vi "testOpenCloseVeriStandConnection.vi"(8 "error in (no error)":errorcluster, 11 "TestCase in":refnum<class "VeriStandTestCaseSystemTests.lvclass">) -> (0 "error out":errorcluster, 3 "TestCase out":refnum<class "VeriStandTestCaseSystemTests.lvclass">)   [LabVIEW 2016, in "VeriStandTestCaseSystemTests.lvclass"]
uses:
  VeriStandTestCaseSystemTests.lvclass
  VeriStandTestUtilities/SystemDefinitionInformation.ctl
  VeriStandTestUtilities/TargetInformation.ctl
  VeriStandTestUtilities/ChassisInformation.ctl
  <vilib>/NI Veristand/Execution/Workspace/WorkspaceAPI.ctl
  NationalInstruments.VeriStand.ClientAPI
  VeriStandTestCase.lvclass
  <vilib>/addons/_JKI Toolkits/VI Tester/TestCase.llb/TestCase.lvclass
  C:/Program Files (x86)/National Instruments/LabVIEW 2016/vi.lib/addons/_JKI Toolkits/VI Tester/TestCase.llb/TestCase.lvclass
  VeriStandTestUtilities/VeriStandTestUtilities.lvlib
  <vilib>/NI VeriStand/Execution/Workspace/NI_VS Workspace ExecutionAPI.lvlib
panel:
  out "WorkspaceManager":T1
  out "System Definition Information":T2
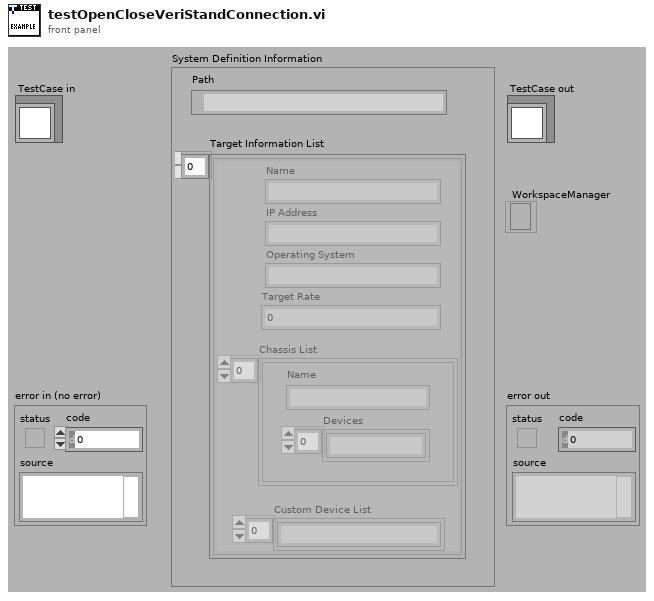
[diagram p1: front panel]
types:
  T1 = typedef "NI_VS Workspace ExecutionAPI.lvlib/WorkspaceAPI.ctl" = refnum<k24>
  T2 = typedef "VeriStandTestUtilities.lvlib/SystemDefinitionInformation.ctl" = cluster{"Path":path, "Target Information List":T3[]}
  T3 = typedef "VeriStandTestUtilities.lvlib/TargetInformation.ctl" = cluster{"Name":string, "IP Address":string, "Operating System":string, "Target Rate":dbl, "Chassis List":T4[], "Custom Device List":string[]}
  T4 = typedef "VeriStandTestUtilities.lvlib/ChassisInformation.ctl" = cluster{"Name":string, "Devices":string[]}
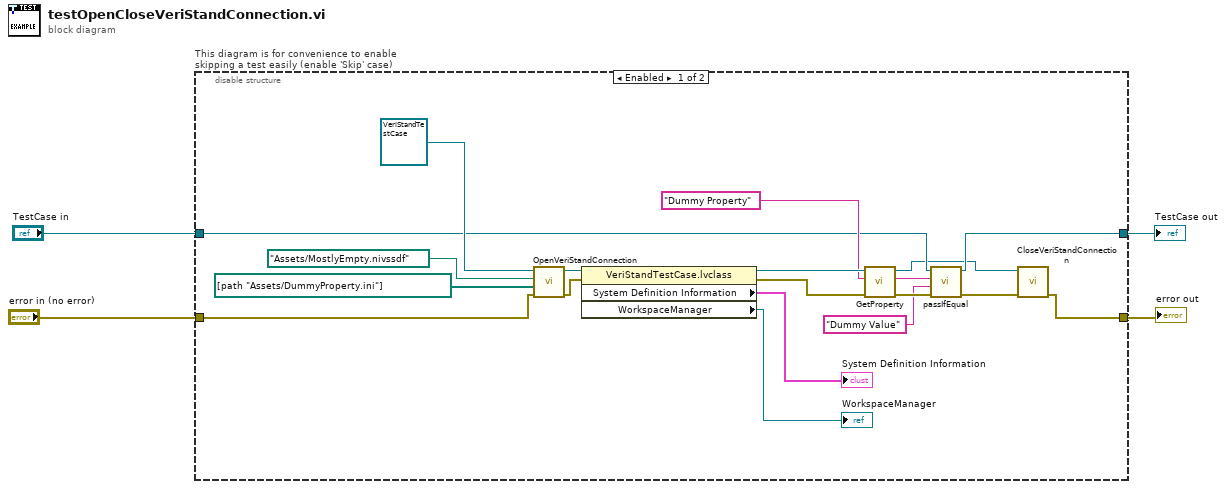
[diagram p0: block diagram]
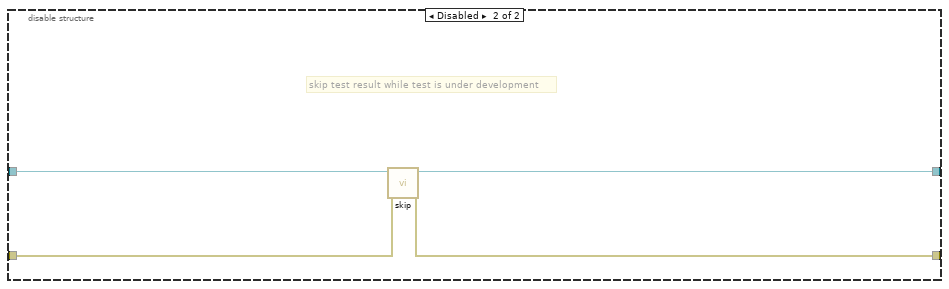
[diagram p2: hidden frame]
diagram:
  n1 = disable-structure "This diagram is for convenience to enable skipping a test easily (enable 'Skip' case)" shown="Enabled" {
    disable-tunnel: "TestCase in" -> [w10 w27]
    disable-tunnel: [w9 w25] -> w1
    disable-tunnel: [w21 w26] -> w3
    disable-tunnel: "error in (no error)" -> [w22 w24]
    frame Enabled {
      n2 = call-dynamic "OpenVeriStandConnection.vi"("error in (no error)"=w22, "overrides files"=path[] [path "Assets/DummyProperty.ini"], "System Definition File"=path "Assets/MostlyEmpty.nivssdf", "VeriStand Test Case in"=refnum<class "VeriStandTestCase.lvclass"> refnum) -> ("error out"=w18:errorcluster, "VeriStand Test Case out"=w19:refnum<class "VeriStandTestCase.lvclass">)  [unwired: 5 in, 1 out]
      n3 = property class="VeriStandTestCase.lvclass"(reference=w19, error in=w18) -> (reference out=w15:refnum<class "VeriStandTestCase.lvclass">, error out=w14:errorcluster, "System Definition Information"=→"System Definition Information":T2, "WorkspaceManager"=→"WorkspaceManager":T1)
      n4 = call "GetProperty.vi"("error in (no error)"=w14, "key"="Dummy Property", "VeriStandTestCase in"=w15) -> ("error out"=w12:errorcluster, "value"=w8:string, "VeriStandTestCase out"=w7:refnum<class "VeriStandTestCase.lvclass">)  [unwired: 6 in]
      n5 = call-dynamic "passIfEqual.vi"("error in (no error)"=w12, "y"="Dummy Value" ("key"), "x"=w8, "TestCase in"=w10) -> ("error out"=w11:errorcluster, "TestCase out"=w9:refnum<class "VeriStandTestCaseSystemTests.lvclass">)  [unwired: 6 in]
      n6 = call-dynamic "CloseVeriStandConnection.vi"("error in (no error)"=w11, "VeriStand Test Case in"=w7) -> ("error out"=w21:errorcluster)  [unwired: 8 in, 1 out]
    }
    frame Disabled {
      # "skip test result while test is under development"
      n7 = call <vilib>:"skip.vi"("error in (no error)"=w24, "TestCase in"=w27) -> ("error out"=w26:errorcluster, "TestCase out"=w25:refnum<class "VeriStandTestCaseSystemTests.lvclass">)  [unwired: 8 in]
    }
  }
  "error out" <- w3
  "TestCase out" <- w1
